vi "Parse-attribute.vi"(8 "error in (no error)":errorcluster, 10 "String in":string, 11 "Offset in":refnum<class "Offset.lvclass">) -> (0 "error out":errorcluster, 1 "Valid attribute?":bool, 2 "Remaining string":string, 3 "Offset out":refnum<class "Offset.lvclass">)   [LabVIEW 2013, in "MaterialCharacterization.lvlib" / "Offset.lvclass"]
uses:
  Offset.lvclass
  Attributes.ctl
  Attribute-ID.ctl
  Attribute-XML.lvclass/Attribute-XML.ctl
  ID.lvclass/ID.ctl
  Coordinate/Coordinate.lvclass/Coordinate.ctl
  Write Attribute.vi
  Write ID-attribute.vi
  Coordinate/Write X.vi
  Coordinate/Write Y.vi
  Attribute-XML.lvclass
  ID.lvclass
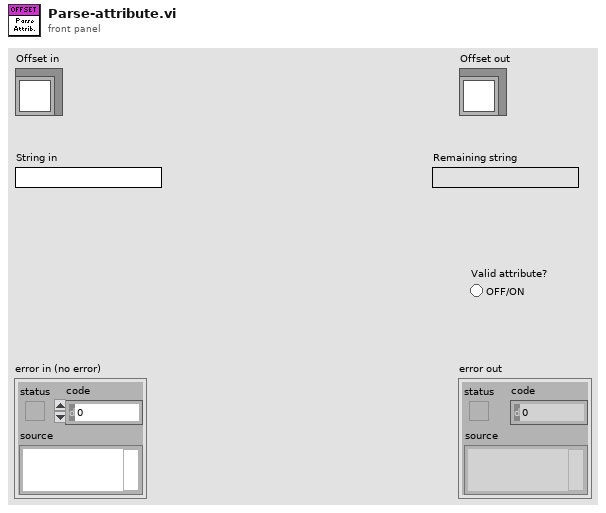
[diagram p1: front panel]
types:
  T1 = typedef "MaterialCharacterization.lvlib/ID.lvclass/Attribute-ID.ctl" = enum16{"FieldOffset", "TransformEnable", "Transform", "Units", "XYCalFactor", "EnableLaser", "JumpDelay", "MarkDelay", "PolyDelay", "LaserOnDelay", "LaserOffDelay", "JumpSpeed", "MarkSpeed", "LaserPowerDelay", "LaserEnableDelay", "LaserPower", "Offset"}
  T2 = typedef "MaterialCharacterization.lvlib/Attribute-XML.lvclass/Attributes.ctl" = enum16{"id"}
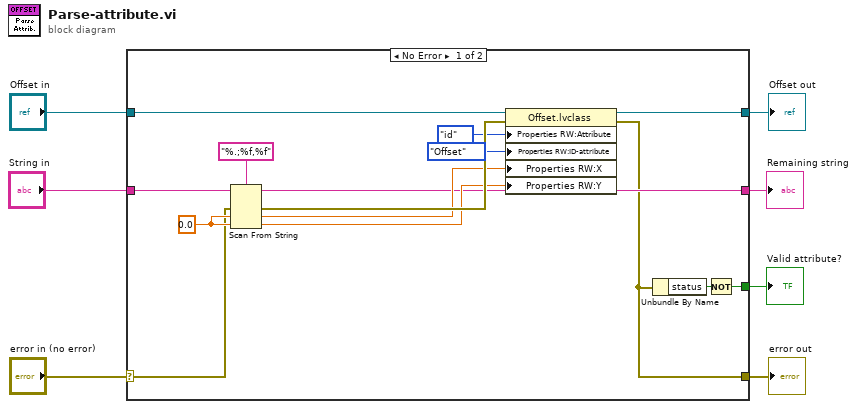
[diagram p0: block diagram]
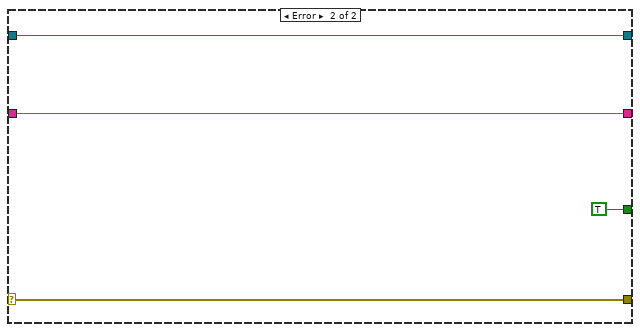
[diagram p2: hidden frame]
diagram:
  n1 = case shown="No Error" "error in (no error)" {
    selector: "error in (no error)" -> [w8 w26]
    tunnel: [w9 w26] -> w6
    tunnel: [w13 w25] -> w4
    tunnel: "Offset in" -> [w14 w25]
    tunnel: "String in" -> [w12 w24]
    tunnel: [w11 w24] -> w2
    tunnel: [w10 TRUE] -> w1
    frame No Error {
      w17 = 0.0 ("default value 2")
      n2 = Scan From String(format string="%.;%f,%f", input string=w12, error in=w8, default 1=w17, default 2=w17) -> (remaining string=w11:string, error out=w20:errorcluster, output 1=w16:dbl, output 2=w15:dbl)  [unwired: 1 in, 1 out]
      n3 = property class="Offset.lvclass"(reference=w14, error in=w20, "Properties RW:Attribute"=Attributes."id" ("Attribute"), "Properties RW:ID-attribute"=Attribute-ID."Offset" ("ID-attribute"), "Properties RW:X"=w16, "Properties RW:Y"=w15) -> (reference out=w13:refnum<class "Offset.lvclass">, error out=w9:errorcluster)
      n4 = Unbundle By Name(w9) -> ("status"=w21:bool)
      n5 = Not(x=w21) -> (.not. x?=w10:bool)
    }
    frame Error {
    }
  }
  "error out" <- w6
  "Offset out" <- w4
  "Remaining string" <- w2
  "Valid attribute?" <- w1
